vi "Modbus Serial Master Example.vi"() -> ()   [LabVIEW 2021]
doc: "An example of the modbus master functionality."
uses:
  API/Wrapper/API Main.lvlib
  Master Function Definition/Read Device ID code.ctl
  Data Model/Device Data Model.lvclass
  API/Master/Modbus Master.lvclass
  API/Wrapper/Create Serial Master.vi
panel:
  in  "serial type":enum16{"RTU", "ASCII"}(ring)
  in  "Serial Resource":refnum<visa-resource-name>
  in  "Stop Button":bool
  in  "Set Holding Registers":bool
  in  "Set Coils":bool
  in  "Fetch Discrete Inputs":bool
  in  "Fetch Input Registers":bool
  in  "Fetch Basic Objects":bool
  out "Basic Objects":string[](array[string])
  out "Status":string
  in  "Disconnect":bool
  in  "Connect":bool
  in  "Holding Registers":u16[](array[numeric])=[0, 0, 0, 0, 0, 0, 0, 0]
  out "Input Registers":u16[](array[numeric])
  in  "Coils":bool[](array[boolean])=[FALSE, FALSE, FALSE, FALSE, FALSE, FALSE, FALSE, FALSE]
  out "Discrete Inputs":bool[](array[boolean])
  # "Coils are the boolean outputs of a modbus device. This example allows you to set the first 8 outputs."
  # "Holding Registers are the integer outputs of a modbus device. This example allows you to set the first 8 outputs."
  # "Modbus devices can also store objects in their memory, which are variable length strings. This example requests the basic level of objects."
  # "Discrete inputs are the boolean inputs of a modbus device. This example allows you to read the first 8 inputs."
  # "Input Registers are the integer inputs of a modbus device. This example allows you to read the first 8 inputs."
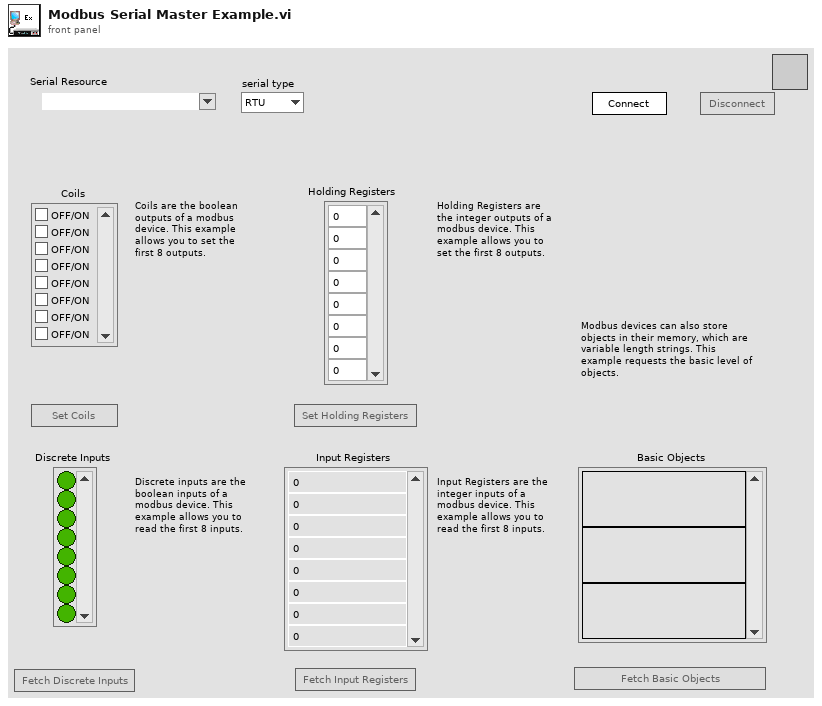
[diagram p1: front panel]
types:
  T1 = enum8{"Enabled", "Disabled", "Disabled and Grayed Out"}
  T2 = typedef "Device Data Model.lvclass/Read Device ID code.ctl" = enum8{"Read Basic", "Read Regular", "Read Extended", "Read Specific"}
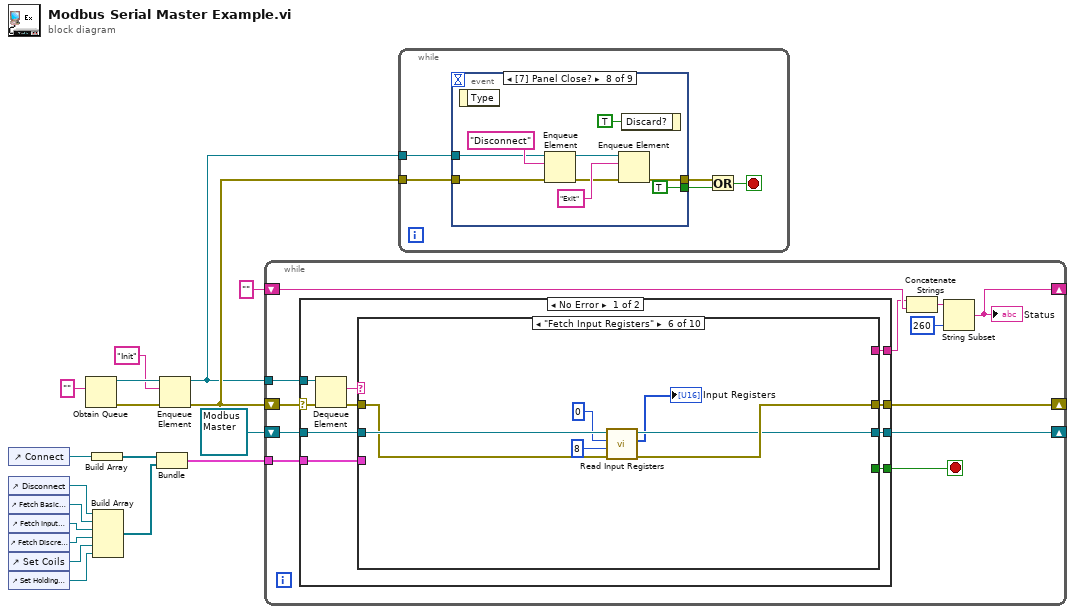
[diagram p0: block diagram]
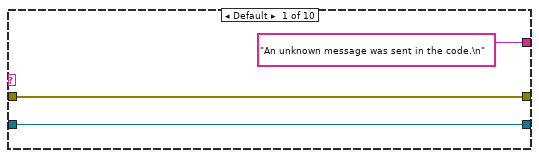
[diagram p2: hidden frame]
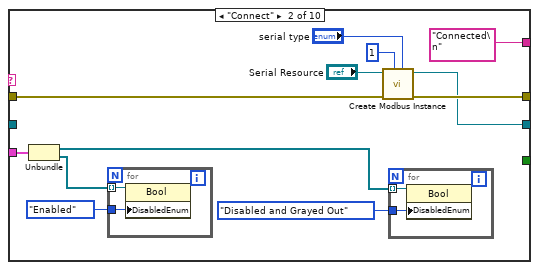
[diagram p3: hidden frame]
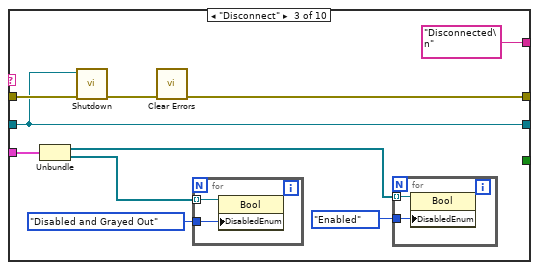
[diagram p4: hidden frame]
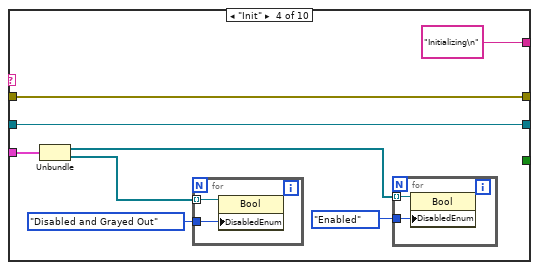
[diagram p5: hidden frame]
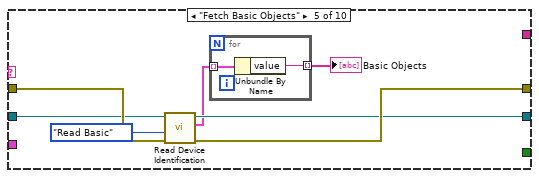
[diagram p6: hidden frame]
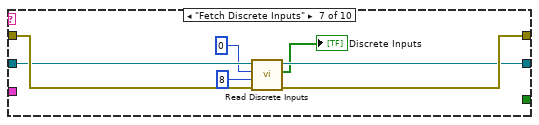
[diagram p7: hidden frame]
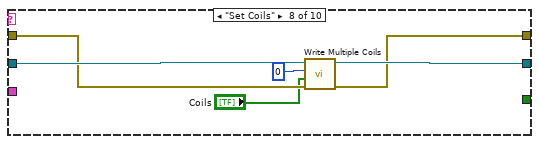
[diagram p8: hidden frame]
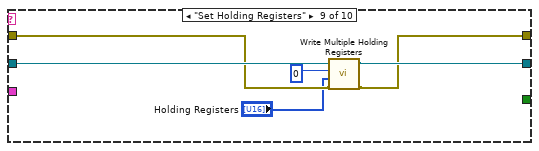
[diagram p9: hidden frame]
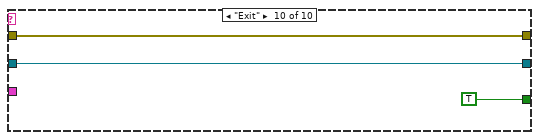
[diagram p10: hidden frame]
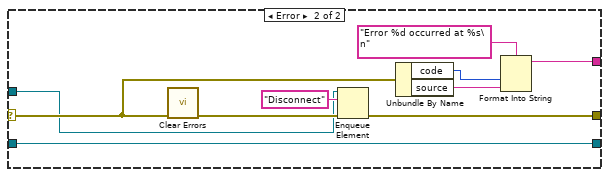
[diagram p11: hidden frame]
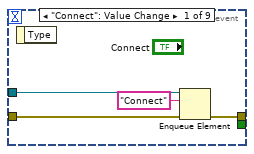
[diagram p12: hidden frame]
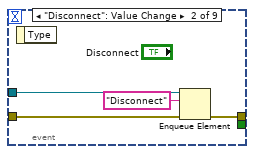
[diagram p13: hidden frame]
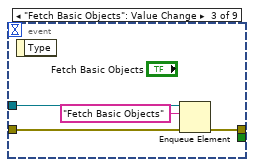
[diagram p14: hidden frame]
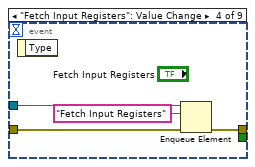
[diagram p15: hidden frame]
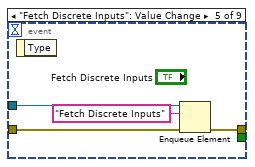
[diagram p16: hidden frame]
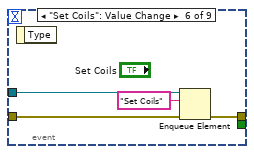
[diagram p17: hidden frame]
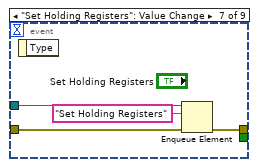
[diagram p18: hidden frame]
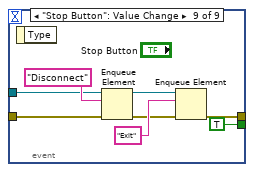
[diagram p19: hidden frame]
diagram:
  n1 = control-ref of="Connect"() -> (w9:refnum<vi>)
  n2 = control-ref of="Disconnect"() -> (w15:refnum<vi>)
  n3 = control-ref of="Fetch Basic Objects"() -> (w14:refnum<vi>)
  n4 = control-ref of="Fetch Input Registers"() -> (w13:refnum<vi>)
  n5 = control-ref of="Fetch Discrete Inputs"() -> (w12:refnum<vi>)
  n6 = control-ref of="Set Coils"() -> (w11:refnum<vi>)
  n7 = control-ref of="Set Holding Registers"() -> (w10:refnum<vi>)
  n8 = Obtain Queue(element data type="") -> (queue out=w4:refnum<queue>, error out=w18:errorcluster)  [unwired: 4 in, 1 out]
  n9 = Build Array(w9) -> (w6:refnum<vi>[])
  n10 = Build Array(w15, w14, w13, w12, w11, w10) -> (w8:refnum<vi>[])
  n11 = Bundle(w6, w8) -> (w7:cluster{refnum<vi>[], refnum<vi>[]})  [unwired: 1 in]
  n12 = Enqueue Element(queue=w4, element="Init", error in (no error)=w18) -> (queue out=w3:refnum<queue>, error out=w5:errorcluster)  [unwired: 1 in, 1 out]
  n13 = while {
    shift-right: [w22] -> _
    shift-left: refnum<class "Modbus Master.lvclass"> refnum ("Modbus Master") -> [w21]
    tunnel: w3 -> [w30]
    shift-right: [w28] -> _
    shift-left: w5 -> [w29]
    shift-right: [w27] -> _
    shift-left: "" ("Status") -> [w24]
    tunnel: w7 -> [w19]
    stop <- w20 stop-if-true
    n14 = case shown="No Error" w29 {
      selector: w29 -> [w39 w131]
      tunnel: w30 -> [w40 w125]
      tunnel: [w36 w132] -> w28
      tunnel: [w33 w128] -> w23
      tunnel: [w35 w124] -> w22
      tunnel: w21 -> [w34 w124]
      tunnel: [w32 _] -> w20
      tunnel: w19 -> [w31 _]
      frame No Error {
        n15 = Dequeue Element(queue=w40, error in (no error)=w39) -> (element=w37:string, error out=w38:errorcluster)  [unwired: 1 in, 2 out]
        n16 = case shown="\"Fetch Input Registers\"" w37 {
          tunnel: w38 -> [w43 w55 w69 w81 w92 w98 w108 w111 w117 w123]
          tunnel: [w43 w54 w65 w81 w91 w101 w107 w112 w118 w123] -> w36
          tunnel: [w42 w53 w67 w80 w89 w100 w105 w113 w119 w122] -> w35
          tunnel: w34 -> [w42 _ w67 w80 w90 w99 w106 w114 w120 w122]
          tunnel: ["An unknown message was sent in the code.\n" "Connected\n" "Disconnected\n" "Initializing\n" _ _ _ _ _ _] -> w33
          tunnel: [_ _ _ _ _ _ _ _ _ TRUE] -> w32
          tunnel: w31 -> [_ w51 w64 w78 _ _ _ _ _ _]
          frame Default {
          }
          frame "Connect" {
            n17 = Unbundle(w51) -> (w49:refnum<vi>[], w50:refnum<vi>[])
            n18 = for {
              tunnel: w50 -> [w57] mode=indexing
              tunnel: T1."Enabled" ("Disabled") -> [w56]
              n19 = property class="Bool"(reference=w57, "DisabledEnum"=w56) -> ()  [unwired: 1 in, 2 out]
            }
            n20 = call-poly "Create Modbus Instance.vi"("serial type"="serial type", "unit ID"=u8 1, "error in"=w55, "VISA resource name"="Serial Resource") -> ("error out"=w54:errorcluster, "serial master instance"=w53:refnum<class "Modbus Master.lvclass">)  [unwired: 6 in]
            n21 = for {
              tunnel: w49 -> [w59] mode=indexing
              tunnel: T1."Disabled and Grayed Out" ("Disabled") -> [w58]
              n22 = property class="Bool"(reference=w59, "DisabledEnum"=w58) -> ()  [unwired: 1 in, 2 out]
            }
          }
          frame "Disconnect" {
            n23 = Unbundle(w64) -> (w62:refnum<vi>[], w63:refnum<vi>[])
            n24 = call-dynamic "Shutdown.vi"("error in (no error)"=w69, "Modbus master in"=w67) -> ("error out"=w68:errorcluster)  [unwired: 9 in]
            n25 = call <vilib>:"Clear Errors.vi"("error in (no error)"=w68) -> ("error out"=w65:errorcluster)  [unwired: 5 in, 1 out]
            n26 = for {
              tunnel: w63 -> [w73] mode=indexing
              tunnel: T1."Disabled and Grayed Out" ("Disabled") -> [w72]
              n27 = property class="Bool"(reference=w73, "DisabledEnum"=w72) -> ()  [unwired: 1 in, 2 out]
            }
            n28 = for {
              tunnel: w62 -> [w71] mode=indexing
              tunnel: T1."Enabled" ("Disabled") -> [w70]
              n29 = property class="Bool"(reference=w71, "DisabledEnum"=w70) -> ()  [unwired: 1 in, 2 out]
            }
          }
          frame "Init" {
            n30 = Unbundle(w78) -> (w76:refnum<vi>[], w77:refnum<vi>[])
            n31 = for {
              tunnel: w77 -> [w85] mode=indexing
              tunnel: T1."Disabled and Grayed Out" ("Disabled") -> [w84]
              n32 = property class="Bool"(reference=w85, "DisabledEnum"=w84) -> ()  [unwired: 1 in, 2 out]
            }
            n33 = for {
              tunnel: w76 -> [w83] mode=indexing
              tunnel: T1."Enabled" ("Disabled") -> [w82]
              n34 = property class="Bool"(reference=w83, "DisabledEnum"=w82) -> ()  [unwired: 1 in, 2 out]
            }
          }
          frame "Fetch Basic Objects" {
            n35 = call-dynamic "Read Device Identification.vi"("error in (no error)"=w92, "read device ID code"=Read_Device_ID_code."Read Basic" ("Read Device ID code"), "Modbus master in"=w90) -> ("error out"=w91:errorcluster, "objects"=w87:cluster{"object ID":u8, "value":string}[], "Modbus master out"=w89:refnum<class "Modbus Master.lvclass">)  [unwired: 6 in]
            n36 = for {
              tunnel: w87 -> [w94] mode=indexing
              tunnel: [w93] -> w86 mode=indexing
              n37 = Unbundle By Name(w94) -> ("value"=w93:string)
            }
            "Basic Objects" <- w86
          }
          frame "Fetch Input Registers" {
            n38 = call-dynamic "Read Input Registers.vi"("error in (no error)"=w98, "number of input registers"=u16 8 ("number of registers"), "starting address"=u16 0, "Modbus master in"=w99) -> ("error out"=w101:errorcluster, "register values"=→"Input Registers":u16[], "Modbus master out"=w100:refnum<class "Modbus Master.lvclass">)  [unwired: 5 in]
          }
          frame "Fetch Discrete Inputs" {
            n39 = call-dynamic "Read Discrete Inputs.vi"("error in (no error)"=w108, "number of discrete inputs"=u16 8 ("number of inputs"), "starting address"=u16 0, "Modbus master in"=w106) -> ("error out"=w107:errorcluster, "discrete input values"=→"Discrete Inputs":bool[], "Modbus master out"=w105:refnum<class "Modbus Master.lvclass">)  [unwired: 5 in]
          }
          frame "Set Coils" {
            n40 = call-dynamic "Write Multiple Coils.vi"("error in (no error)"=w111, "coil values"="Coils", "starting address"=u16 0, "Modbus master in"=w114) -> ("error out"=w112:errorcluster, "Modbus master out"=w113:refnum<class "Modbus Master.lvclass">)  [unwired: 6 in]
          }
          frame "Set Holding Registers" {
            n41 = call-dynamic "Write Multiple Holding Registers.vi"("error in (no error)"=w117, "holding register values"="Holding Registers", "starting address"=u16 0, "Modbus master in"=w120) -> ("error out"=w118:errorcluster, "Modbus master out"=w119:refnum<class "Modbus Master.lvclass">)  [unwired: 6 in]
          }
          frame "Exit" {
          }
        }
      }
      frame Error {
        n42 = call <vilib>:"Clear Errors.vi"("error in (no error)"=w131) -> ("error out"=w133:errorcluster)  [unwired: 5 in, 1 out]
        n43 = Enqueue Element(queue=w125, element="Disconnect", error in (no error)=w133) -> (error out=w132:errorcluster)  [unwired: 1 in, 2 out]
        n44 = Unbundle By Name(w131) -> ("code"=w130:i32, "source"=w129:string)
        n45 = Format Into String(format string="Error %d occurred at %s\n", w130, w129) -> (resulting string=w128:string)  [unwired: 2 in, 1 out]
      }
    }
    n46 = Concatenate Strings(w23, w24) -> (w25:string)
    n47 = String Subset(string=w25, length (rest)=260 ("length (rest)")) -> (substring=w27:string)  [unwired: 1 in]
    "Status" <- w27
  }
  n48 = while {
    tunnel: w5 -> [w138]
    tunnel: w3 -> [w137]
    stop <- w134 stop-if-true
    n49 = event shown="[7] Panel Close?" {
      selector: _ -> [_ _ _ _ _ _ _ _ _]
      dyn-events: _ -> [_ _ _ _ _ _ _ _ _]
      timeout: _ -> [_ _ _ _ _ _ _ _ _]
      tunnel: w138 -> [w142 w146 w150 w154 w158 w162 w166 w172 w181]
      tunnel: [w141 w145 w149 w153 w157 w161 w165 w167 w176] -> w136
      tunnel: w137 -> [w140 w144 w148 w152 w156 w160 w164 w169 w178]
      tunnel: [_ _ _ _ _ _ _ TRUE ("Discard?") TRUE ("Discard?")] -> w135
      event "Connect": Value Change {
        n50 = event-data() -> ()  [unwired: 1 in, 1 out]
        n51 = Enqueue Element(queue=w140, element="Connect", error in (no error)=w142) -> (error out=w141:errorcluster)  [unwired: 1 in, 2 out]
      }
      event "Disconnect": Value Change {
        n52 = event-data() -> ()  [unwired: 1 in, 1 out]
        n53 = Enqueue Element(queue=w144, element="Disconnect", error in (no error)=w146) -> (error out=w145:errorcluster)  [unwired: 1 in, 2 out]
      }
      event "Fetch Basic Objects": Value Change {
        n54 = event-data() -> ()  [unwired: 1 in, 1 out]
        n55 = Enqueue Element(queue=w148, element="Fetch Basic Objects", error in (no error)=w150) -> (error out=w149:errorcluster)  [unwired: 1 in, 2 out]
      }
      event "Fetch Input Registers": Value Change {
        n56 = event-data() -> ()  [unwired: 1 in, 1 out]
        n57 = Enqueue Element(queue=w152, element="Fetch Input Registers", error in (no error)=w154) -> (error out=w153:errorcluster)  [unwired: 1 in, 2 out]
      }
      event "Fetch Discrete Inputs": Value Change {
        n58 = event-data() -> ()  [unwired: 1 in, 1 out]
        n59 = Enqueue Element(queue=w156, element="Fetch Discrete Inputs", error in (no error)=w158) -> (error out=w157:errorcluster)  [unwired: 1 in, 2 out]
      }
      event "Set Coils": Value Change {
        n60 = event-data() -> ()  [unwired: 1 in, 1 out]
        n61 = Enqueue Element(queue=w160, element="Set Coils", error in (no error)=w162) -> (error out=w161:errorcluster)  [unwired: 1 in, 2 out]
      }
      event "Set Holding Registers": Value Change {
        n62 = event-data() -> ()  [unwired: 1 in, 1 out]
        n63 = Enqueue Element(queue=w164, element="Set Holding Registers", error in (no error)=w166) -> (error out=w165:errorcluster)  [unwired: 1 in, 2 out]
      }
      event Panel Close? {
        n64 = event-data() -> ()  [unwired: 1 in, 1 out]
        n65 = Enqueue Element(queue=w169, element="Disconnect", error in (no error)=w172) -> (queue out=w170:refnum<queue>, error out=w168:errorcluster)  [unwired: 1 in, 1 out]
        n66 = Enqueue Element(queue=w170, element="Exit", error in (no error)=w168) -> (error out=w167:errorcluster)  [unwired: 1 in, 2 out]
        n67 = event-data("Discard?"=TRUE) -> ()  [unwired: 1 in, 1 out]
      }
      event "Stop Button": Value Change {
        n68 = event-data() -> ()  [unwired: 1 in, 1 out]
        n69 = Enqueue Element(queue=w178, element="Disconnect", error in (no error)=w181) -> (queue out=w179:refnum<queue>, error out=w177:errorcluster)  [unwired: 1 in, 1 out]
        n70 = Enqueue Element(queue=w179, element="Exit", error in (no error)=w177) -> (error out=w176:errorcluster)  [unwired: 1 in, 2 out]
      }
    }
    n71 = Or(x=w136, y=w135) -> (x .or. y?=w134:bool)
  }
